vi "Build.vi"(6 "Assembly Type":string, 8 "Position":i32, 9 "XYZTheta":dbl[](array[numeric]), 10 "text file":dbl[][](array[numeric]), 11 "Sensor Dispense in":refnum<class "Sensor Dispense.lvclass">) -> (3 "Sensor Dispense out":refnum<class "Sensor Dispense.lvclass">)   [LabVIEW 2021, in "Sensor Dispense.lvclass"]
uses:
  Projects/Sensor Dispense.lvclass
  C:/Users/HEP/Documents/GitHub/Gantry/UCSB-Gantry-HEP-main/Classes/Routine/Dispense/Dispense.lvclass
  Projects/Sensor Dispense.lvclass/Sensor Dispense.ctl
  <vilib>/Analysis/coordinate.llb/2D Cartesian Coordinate Rotation (Scalar).vi
  <vilib>/Analysis/NI_AALPro.lvlib
panel:
  out "CW/CCW":dbl[](array[numeric])
  out "CW/CCW":dbl[](array[numeric])
  out "endpoints 2":dbl[][](array[numeric])
  out "endpoints":dbl[][](array[numeric])
  out "data":T1(array[cluster])
  out "cell count":dbl[](array[numeric])
  out "centers":dbl[][](array[numeric])
  # "[x1,y1,x2,y2]"
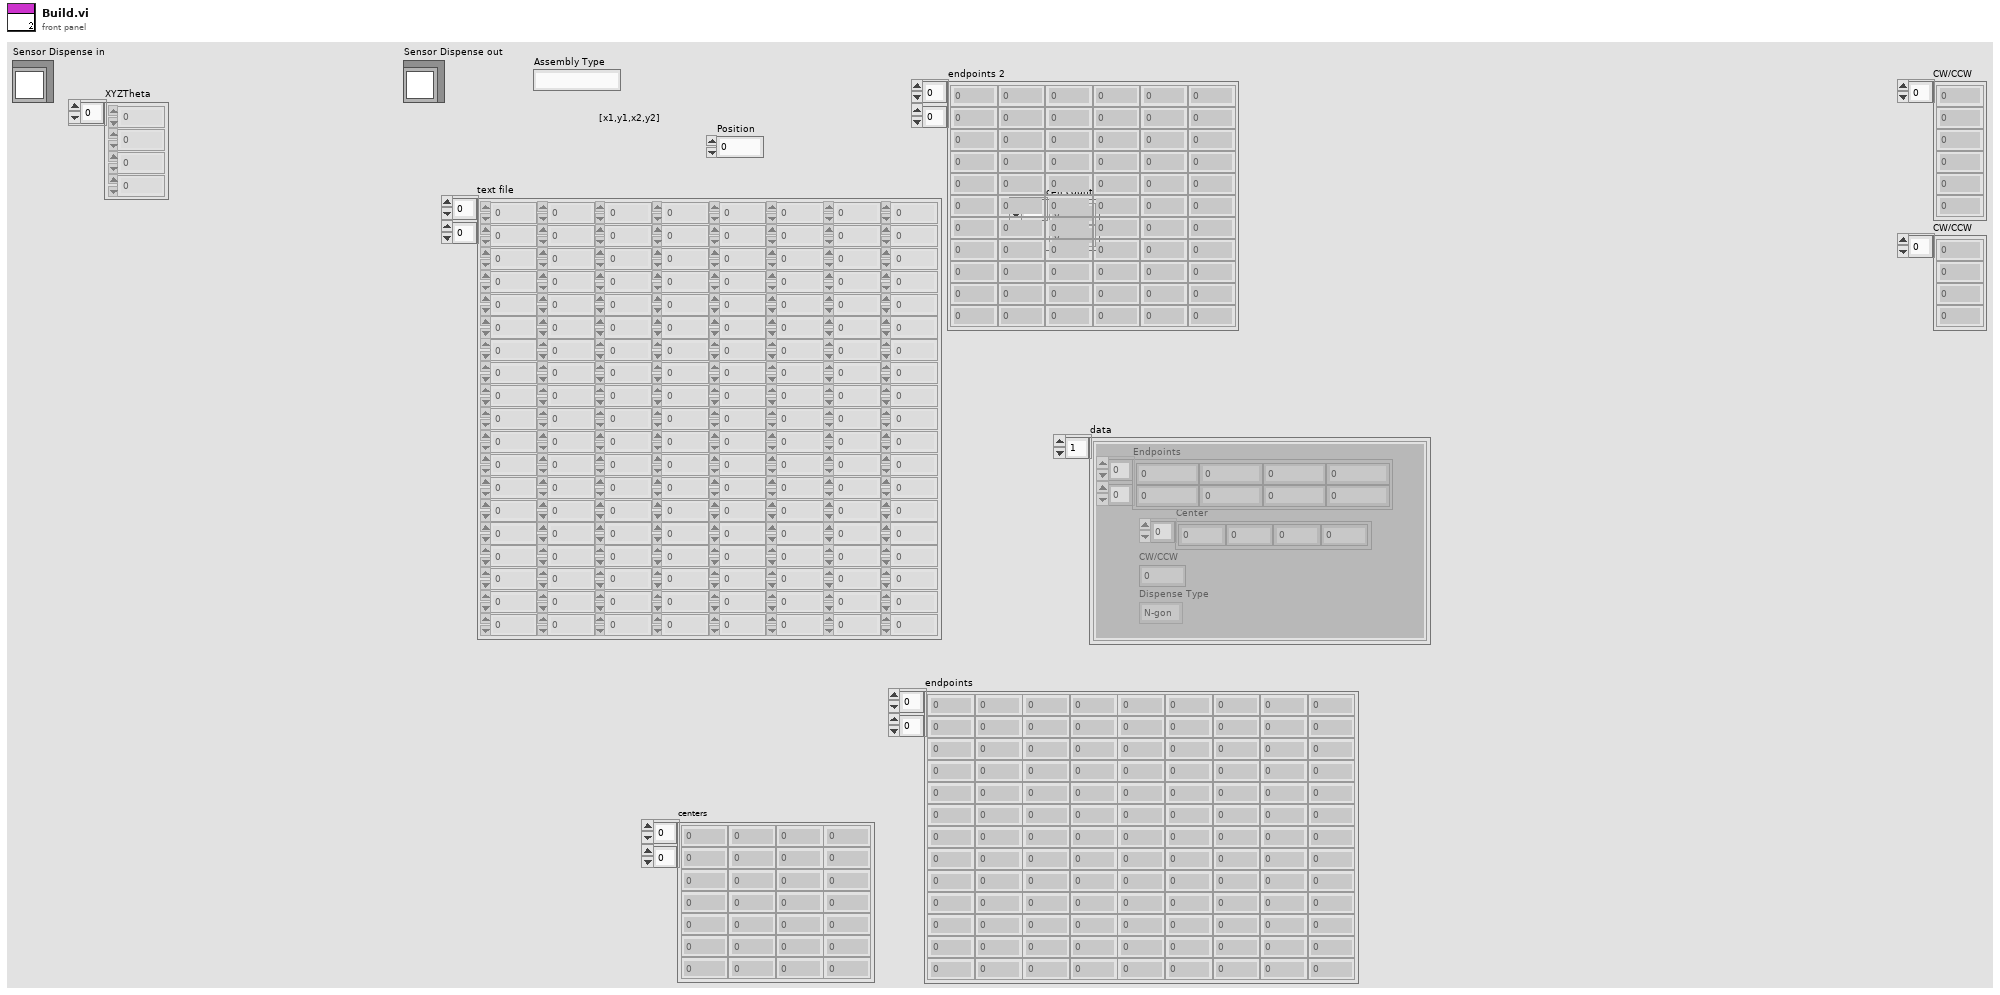
[diagram p1: front panel]
types:
  T1 = cluster{"Endpoints":dbl[][], "Center":dbl[], "CW/CCW":dbl, "Dispense Type":enum16{"N-gon", "Square", "Arc", "Dot", "Line", "Circle"}}[]
  T2 = enum16{"N-gon", "Square", "Arc", "Dot", "Line", "Circle"}
  T3 = cluster{"Endpoints":dbl[][], "Center":dbl[], "CW/CCW":dbl, "Dispense Type":enum16{"N-gon", "Square", "Arc", "Dot", "Line", "Circle"}}
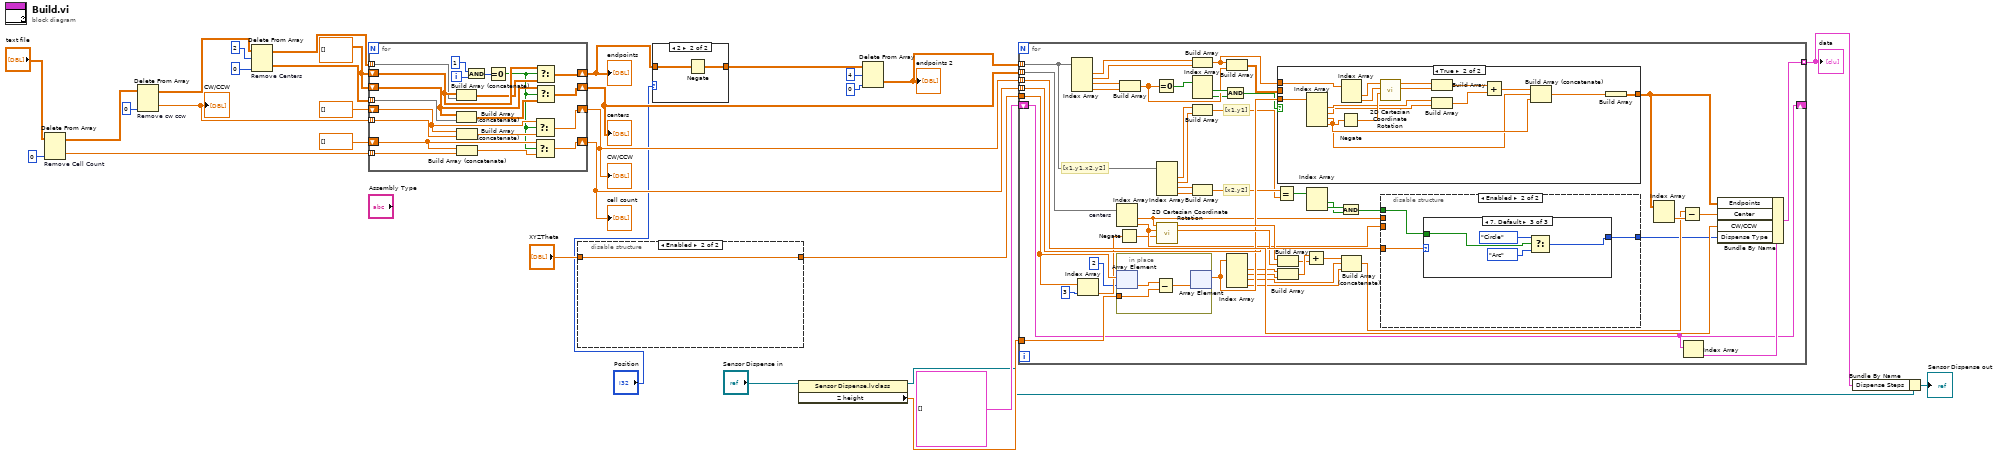
[diagram p0: block diagram]
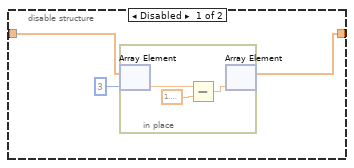
[diagram p3: hidden frame]
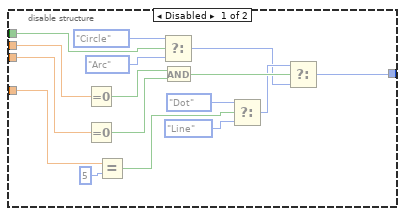
[diagram p4: hidden frame]
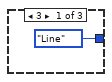
[diagram p5: hidden frame]
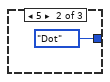
[diagram p6: hidden frame]
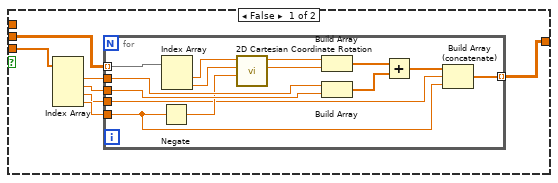
[diagram p7: hidden frame]
diagram:
  w28 = dbl[][] []
  n1 = Delete From Array "Remove Cell Count"(array="text file", index (col)=0) -> (deleted portion=w22:dbl[], array with subset deleted=w24:dbl[][])  [unwired: 2 in]
  n2 = Delete From Array "Remove cw ccw"(array=w24, index (col)=0 ("disabled index (col)")) -> (deleted portion=w5:dbl[], array with subset deleted=w21:dbl[][])  [unwired: 2 in]
  "CW/CCW" <- w5
  n3 = Delete From Array "Remove Centers"(array=w21, length=2, index (col)=0) -> (deleted portion=w17:dbl[][], array with subset deleted=w18:dbl[][])  [unwired: 1 in]
  n4 = for {
    tunnel: w18 -> [w47] mode=indexing
    shift-right: [w45] -> w1
    shift-left: w28 -> [w48]
    tunnel: w17 -> [w44] mode=indexing
    shift-right: [w41] -> w29
    shift-left: w28 -> [w42]
    tunnel: w22 -> [w40] mode=indexing
    shift-right: [w37] -> w26
    shift-left: dbl[] [] -> [w39]
    shift-right: [w32] -> w4
    shift-left: dbl[] [] -> [w35]
    tunnel: w5 -> [w36] mode=indexing
    i -> [w50]
    n5 = Build Array (concatenate)(w48, w47) -> (w46:dbl[][])
    n6 = Build Array (concatenate)(w42, w44) -> (w43:dbl[][])
    n7 = Build Array (concatenate)(w35, w36) -> (w34:dbl[])
    n8 = Build Array (concatenate)(w39, w40) -> (w38:dbl[])
    n9 = And(x=1, y=w50) -> (x .and. y?=w49:i32)
    n10 = Equal To 0?(x=w49) -> (x = 0?=w33:bool)
    n11 = Select(t=w35, s=w33, f=w34) -> (s? t:f=w32:dbl[])
    n12 = Select(t=w39, s=w33, f=w38) -> (s? t:f=w37:dbl[])
    n13 = Select(t=w48, s=w33, f=w46) -> (s? t:f=w45:dbl[][])
    n14 = Select(t=w42, s=w33, f=w43) -> (s? t:f=w41:dbl[][])
  }
  "centers" <- w29
  "cell count" <- w26
  "endpoints" <- w1
  "CW/CCW" <- w4
  n15 = disable-structure shown="Enabled" {
    disable-tunnel: "XYZTheta" -> [w54 w58]
    disable-tunnel: [w52 w58] -> w7
    frame Disabled {
      n16 = in-place {
        n17 = in-place-array #1(w54, 3) -> (w57:dbl)
        n18 = Subtract(x=w57, y=1.5707963267948966) -> (x-y=w55:dbl)
        n19 = in-place-array #1(w55) -> (w52:dbl[])  [unwired: 1 out]
      }
    }
    frame Enabled {
    }
  }
  n20 = case shown="2" "Position" {
    tunnel: [w59 w61] -> w2
    tunnel: w1 -> [w59 w60]
    frame 1, Default {
    }
    frame 2 {
      n21 = Negate(x=w60) -> (-x=w61:dbl[][])
    }
  }
  n22 = property class="Sensor Dispense.lvclass"(reference="Sensor Dispense in") -> (reference out=w14:refnum<class "Sensor Dispense.lvclass">, "Z height"=w31:dbl)  [unwired: 1 in, 1 out]
  n23 = Delete From Array(array=w2, length=4, index (col)=0 ("disabled index (col)")) -> (deleted portion=w9:dbl[][])  [unwired: 1 in, 1 out]
  "endpoints 2" <- w9
  n24 = for {
    tunnel: w9 -> [w75] mode=indexing
    tunnel: w7 -> [w85]
    tunnel: w31 -> [w112]
    tunnel: w29 -> [w111] mode=indexing
    tunnel: w4 -> [w110] mode=indexing
    tunnel: w26 -> [w109] mode=indexing
    shift-right: [w94] -> _
    shift-left: T1 [] ("Dispense Steps") -> [w94]
    tunnel: [w108] -> w13 mode=indexing
    # "[x2,y2]"
    # "[x1,y1]"
    # "[x1,y1,x2,y2]"
    n25 = Index Array(array=w75) -> (element #1=w73:dbl, element #2=w72:dbl, element #3=w71:dbl, element #4=w70:dbl)  [unwired: 4 in]
    n26 = Index Array(array=w85, index=3) -> (element=w84:dbl)
    n27 = Index Array "centers"(array=w111) -> (element #1=w97:dbl, element #2=w96:dbl)  [unwired: 2 in]
    n28 = in-place {
      in-place-border: w112 -> [w139]
      n29 = in-place-array #2(w85, 2) -> (w140:dbl)
      n30 = Subtract(x=w140, y=w139) -> (x-y=w138:dbl)
      n31 = in-place-array #2(w138) -> (w105:dbl[])  [unwired: 1 out]
    }
    n32 = Negate(x=w84) -> (-x=w83:dbl)
    n33 = Build Array(w71, w70) -> (w67:dbl[])
    n34 = Equal To 0?(x=w67) -> (x = 0?=w66:bool[])
    n35 = Index Array(array=w75) -> (element #1=w81:dbl, element #2=w80:dbl, element #3=w93:dbl, element #4=w92:dbl)  [unwired: 4 in]
    n36 = call-poly <vilib>:"2D Cartesian Coordinate Rotation.vi"("theta"=w83, "y"=w96, "x"=w97) -> ("y out"=w106:dbl, "x out"=w107:dbl)  [unwired: 6 in, 1 out]
    n37 = Build Array(w73, w72) -> (w63:dbl[])
    n38 = Index Array(array=w66) -> (element #1=w68:bool, element #2=w64:bool)  [unwired: 2 in]
    n39 = Build Array(w81, w80) -> (w90:dbl[])
    n40 = Build Array(w93, w92) -> (w91:dbl[])
    n41 = And(x=w68, y=w64) -> (x .and. y?=w65:bool)
    n42 = Build Array(w63, w67) -> (w69:dbl[][])
    n43 = Index Array(array=w105) -> (element #1=w104:dbl, element #2=w101:dbl, element #3=w99:dbl, element #4=w98:dbl)  [unwired: 4 in]
    n44 = Equal?(x=w91, y=w90) -> (x = y?=w89:bool[])
    n45 = case shown="True" w65 {
      tunnel: w105 -> [w147 w174]
      tunnel: [w146 w162] -> w79
      tunnel: w69 -> [w145 _]
      tunnel: w63 -> [_ w177]
      frame False {
        n46 = Index Array(array=w147) -> (element #1=w144:dbl, element #2=w143:dbl, element #3=w141:dbl, element #4=w142:dbl)  [unwired: 4 in]
        n47 = for {
          tunnel: w145 -> [w161] mode=indexing
          tunnel: w144 -> [w158]
          tunnel: w143 -> [w157]
          tunnel: [w148] -> w146 mode=indexing
          tunnel: w142 -> [w149]
          tunnel: w141 -> [w150]
          n48 = Negate(x=w149) -> (-x=w152:dbl)
          n49 = Index Array(array=w161) -> (element #1=w160:dbl, element #2=w159:dbl)  [unwired: 2 in]
          n50 = call-poly <vilib>:"2D Cartesian Coordinate Rotation.vi"("theta"=w152, "y"=w159, "x"=w160) -> ("y out"=w155:dbl, "x out"=w156:dbl)  [unwired: 6 in, 1 out]
          n51 = Build Array(w156, w155) -> (w154:dbl[])
          n52 = Build Array(w158, w157) -> (w153:dbl[])
          n53 = Add(x=w154, y=w153) -> (x+y=w151:dbl[])
          n54 = Build Array (concatenate)(w151, w150, w149) -> (w148:dbl[])
        }
      }
      frame True {
        n55 = Index Array(array=w174) -> (element #1=w170:dbl, element #2=w169:dbl, element #3=w165:dbl, element #4=w166:dbl)  [unwired: 4 in]
        n56 = Negate(x=w166) -> (-x=w173:dbl)
        n57 = Index Array(array=w177) -> (element #1=w176:dbl, element #2=w175:dbl)  [unwired: 2 in]
        n58 = call-poly <vilib>:"2D Cartesian Coordinate Rotation.vi"("theta"=w173, "y"=w175, "x"=w176) -> ("y out"=w171:dbl, "x out"=w172:dbl)  [unwired: 6 in, 1 out]
        n59 = Build Array(w172, w171) -> (w167:dbl[])
        n60 = Build Array(w170, w169) -> (w168:dbl[])
        n61 = Add(x=w167, y=w168) -> (x+y=w164:dbl[])
        n62 = Build Array (concatenate)(w164, w165, w166) -> (w163:dbl[])
        n63 = Build Array(w163) -> (w162:dbl[][])
      }
    }
    n64 = Build Array(w107, w106) -> (w102:dbl[])
    n65 = Build Array(w104, w101) -> (w103:dbl[])
    n66 = Add(x=w103, y=w102) -> (x+y=w100:dbl[])
    n67 = Index Array(array=w89) -> (element #1=w87:bool, element #2=w88:bool)  [unwired: 2 in]
    n68 = And(x=w88, y=w87) -> (x .and. y?=w86:bool)
    n69 = Build Array (concatenate)(w100, w99, w98) -> (w77:dbl[])
    n70 = disable-structure shown="Enabled" {
      disable-tunnel: w109 -> [w128 w131]
      disable-tunnel: w97 -> [w125 _]
      disable-tunnel: w96 -> [w124 _]
      disable-tunnel: w86 -> [w117 w130]
      disable-tunnel: [w113 w129] -> w74
      frame Disabled {
        n71 = Equal To 0?(x=w125) -> (x = 0?=w126:bool)
        n72 = Equal To 0?(x=w124) -> (x = 0?=w127:bool)
        n73 = Equal?(x=w128, y=5) -> (x = y?=w120:bool)
        n74 = Select(t=T2."Circle" ("Dispense Type"), s=w117, f=T2."Arc" ("Dispense Type")) -> (s? t:f=w114:T2)
        n75 = And(x=w126, y=w127) -> (x .and. y?=w116:bool)
        n76 = Select(t=T2."Dot" ("Dispense Type"), s=w120, f=T2."Line" ("Dispense Type")) -> (s? t:f=w115:T2)
        n77 = Select(t=w115, s=w116, f=w114) -> (s? t:f=w113:T2)
      }
      frame Enabled {
        n78 = case shown="7, Default" w131 {
          tunnel: w130 -> [_ _ w135]
          tunnel: [T2."Line" ("Dispense Type") T2."Dot" ("Dispense Type") w134] -> w129
          frame 3 {
          }
          frame 5 {
          }
          frame 7, Default {
            n79 = Select(t=T2."Circle" ("Dispense Type"), s=w135, f=T2."Arc" ("Dispense Type")) -> (s? t:f=w134:T2)
          }
        }
      }
    }
    n80 = Index Array(array=w79) -> (element=w78:dbl[])  [unwired: 2 in]
    n81 = Subtract(x=w77, y=w78) -> (x-y=w76:dbl[])
    n82 = Index Array(array=w94) -> (element=w95:T3)  [unwired: 1 in]
    n83 = Bundle By Name(cluster=w95, "Endpoints"=w79, "Center"=w76, "CW/CCW"=w110, "Dispense Type"=w74) -> (w108:T3)
  }
  "data" <- w13
  n84 = Bundle By Name(cluster=w14, "Dispense Steps"=w13) -> (→"Sensor Dispense out":refnum<class "Sensor Dispense.lvclass">)
